vi "Check for Undeploy.vi"(9 "Histogram Data":dbl[](array[numeric]), 11 "Histogram In":cluster{"Array":dbl[], dbl[]}) -> (2 "Histogram Out":cluster{"Array":dbl[], dbl[]})   [LabVIEW 2012]
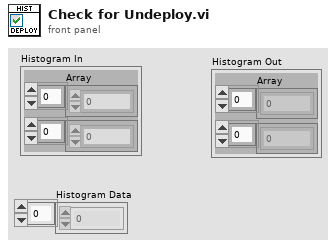
[diagram p1: front panel]
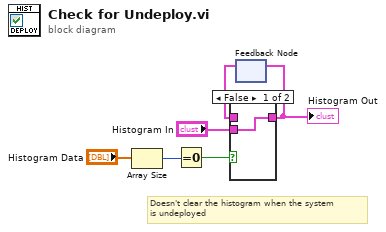
[diagram p0: block diagram]
diagram:
  # "Doesn't clear the histogram when the system\nis undeployed"
  n1 = Array Size(array="Histogram Data") -> (size(s)=w2:i32)
  n2 = Equal To 0?(x=w2) -> (x = 0?=w3:bool)
  n3 = feedback #1() -> (w6:cluster{"Array":dbl[], dbl[]})  [unwired: 1 in]
  n4 = case shown="False" w3 {
    tunnel: "Histogram In" -> [w7 _]
    tunnel: [w7 w8] -> w5
    tunnel: w6 -> [_ w8]
    frame False {
    }
    frame True {
    }
  }
  "Histogram Out" <- w5
  n5 = feedback-in #1(w5) -> ()
